vi "WSVCAP SHL Host TL I2C Read - Single Device.vi"(0 "Bytes to Read (1-4)":u8=4 min=1 max=4 step=1, 5 "Sub Address [U8]":u8=191 format="%.0x", 11 "error in":errorcluster, 12 "DUT":T2, 13 "Device":T1, 14 "Log (T)":bool=TRUE) -> (4 "Device Data":u8[](array[numeric]) format="%.0x", 15 "error out":errorcluster)   [LabVIEW 2012]
uses:
  Type Defs/WSVCAP SHL DUT Number Enum.ctl
  Type Defs/WSVCAP SHL I2C Device Enum.ctl
panel:
  out "C3:1-16 Read Data [U8]":u8[][](array[numeric]) format="%.0x"
  out "Socket Mask [U64]":u64=1 format="%016x"
  out "C2:1-16 Read Data [U8]":u8[][](array[numeric]) format="%.0x"
  out "C1:1-16 Read Data [U8]":u8[][](array[numeric]) format="%.0x"
  out "Data Headers":u8[](array[numeric])=[1, 2, 3, 4, 5, 6, 7, 8, 9, 10, 11, 12, 12, 14, 15, 16]
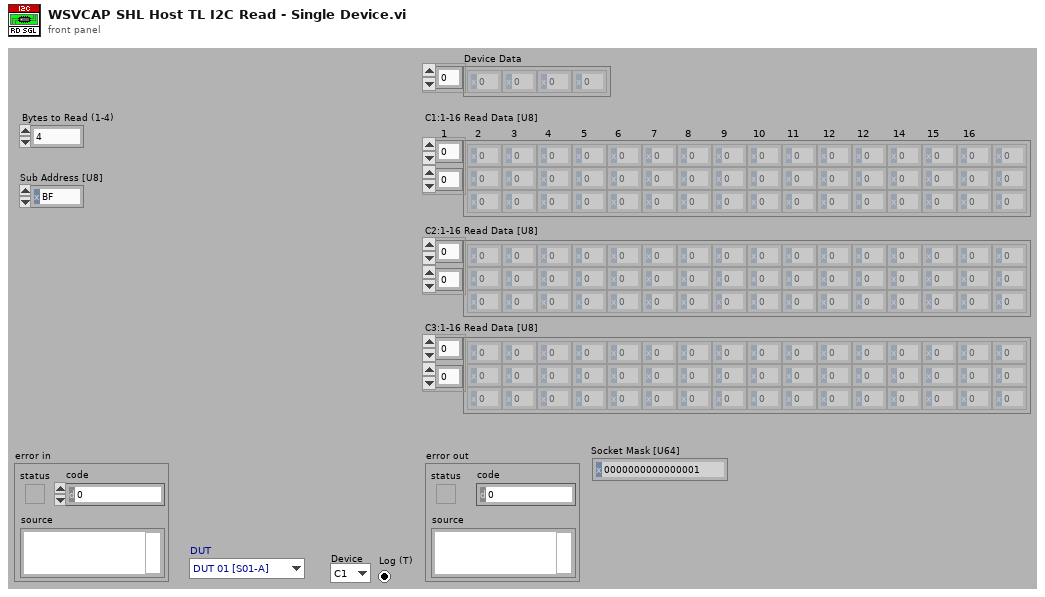
[diagram p1: front panel]
types:
  T1 = typedef "WSVCAP SHL I2C Device Enum.ctl" = enum16{"C1", "C2", "C3"}
  T2 = typedef "WSVCAP SHL DUT Number Enum.ctl" = enum16{"DUT 01 [S01-A]", "DUT 02 [S02-B]", "DUT 03 [S03-C]", "DUT 04 [S04-D]", "DUT 05 [S05-E]", "DUT 06 [S06-F]", "DUT 07 [S07-G]", "DUT 08 [S08-H]", "DUT 09 [S09-I]", "DUT 10 [S10-J]", "DUT 11 [S11-K]", "DUT 12 [S12-L]", "DUT 13 [S13-M]", "DUT 14 [S14-N]", "DUT 15 [S15-O]", "DUT 16 [S16-P]"}
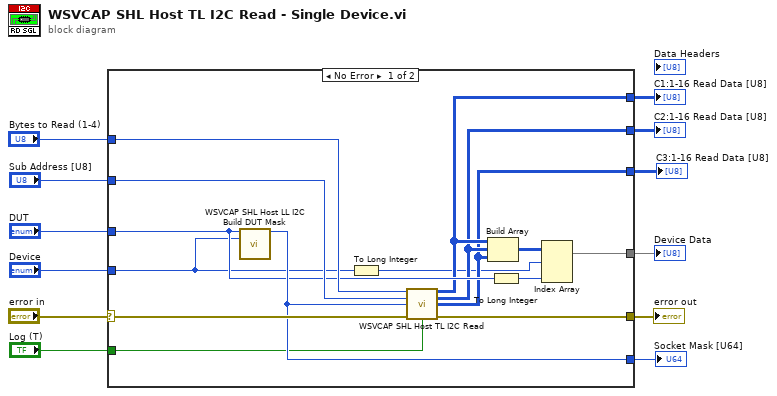
[diagram p0: block diagram]
diagram:
  n1 = case shown="No Error" "error in" {
    selector: "error in" -> [w26 w28]
    tunnel: [w27 w28] -> w12
    tunnel: "Bytes to Read (1-4)" -> [w25 _]
    tunnel: "Sub Address [U8]" -> [w24 _]
    tunnel: "DUT" -> [w21 _]
    tunnel: [w23 _] -> w7
    tunnel: "Device" -> [w14 _]
    tunnel: [w19 _] -> w5
    tunnel: [w18 _] -> w4
    tunnel: [w22 _] -> w3
    tunnel: "Log (T)" -> [w20 _]
    tunnel: [w17 _] -> w1
    frame No Error {
      n2 = call "WSVCAP SHL Host LL I2C Build DUT Mask.vi"("DUT"=w21, "Device"=w14) -> ("Socket Mask [U64]"=w23:u64)  [unwired: 11 in, 2 out]
      n3 = To Long Integer(number=w14) -> (32bit integer=w13:i32)
      n4 = call "WSVCAP SHL Host TL I2C Read.vi"("Bytes to Read"=w25, "Sub Address [U8]"=w24, "Socket Mask [U64]"=w23, "error in"=w26, "Log (T)"=w20) -> ("C1 Read Data Out"=w19:u8[][], "C2 Read Data Out"=w18:u8[][], "C3 Read Data Out"=w17:u8[][], "error out"=w27:errorcluster)  [unwired: 7 in]
      n5 = Build Array(w19, w18, w17) -> (w16:u8[][][])
      n6 = To Long Integer(number=w21) -> (32bit integer=w15:i32)
      n7 = Index Array(array=w16, index (dim 0)=w13, index (dim 2)=w15) -> (element=w22:u8[])  [unwired: 1 in]
    }
    frame Error {
    }
  }
  "error out" <- w12
  "Socket Mask [U64]" <- w7
  "C1:1-16 Read Data [U8]" <- w5
  "C2:1-16 Read Data [U8]" <- w4
  "Device Data" <- w3
  "C3:1-16 Read Data [U8]" <- w1
